vi "TcA03-003_MutualExclusionWhenModifyingClassAttributes.vi"(1 "Input buffer":T3="1", 3 "Invocation info":T2, 5 "error in (no error)":errorcluster, 6 "Add log to result?":bool) -> (16 "Test Data":T1 {"Numeric Measurement" format="%.2f"}, 19 "error out":errorcluster)   [LabVIEW 2020]
doc: "Test case template."
uses:
  Shared/Support_InputBuffer.ctl
  Shared/Support_InvocationInfo.ctl
  Shared/Support_TestData.ctl
  TestClasses/G#BaseClass1_class/G#BaseClass1.lvclass
  TestClasses/G#BaseClass2_class/G#BaseClass2.lvclass
  <vilib>/addons/_AddQ/G#Object/G#Object.lvclass
  TestClasses/G#SubClass2_class/G#SubClass2.lvclass
  TestClasses/G#SubClass1_class/G#SubClass1.lvclass
panel:
  in  "Test name":string="TcA03-003 Mutual Exclusion When Modifying Class Attributes"
  out "Test result":bool
  out "Result":string
  # "Verify that class attributes can be modified and\naccessed , one will be mutual excluded\nand forced to wait."
  # "Sub test case"
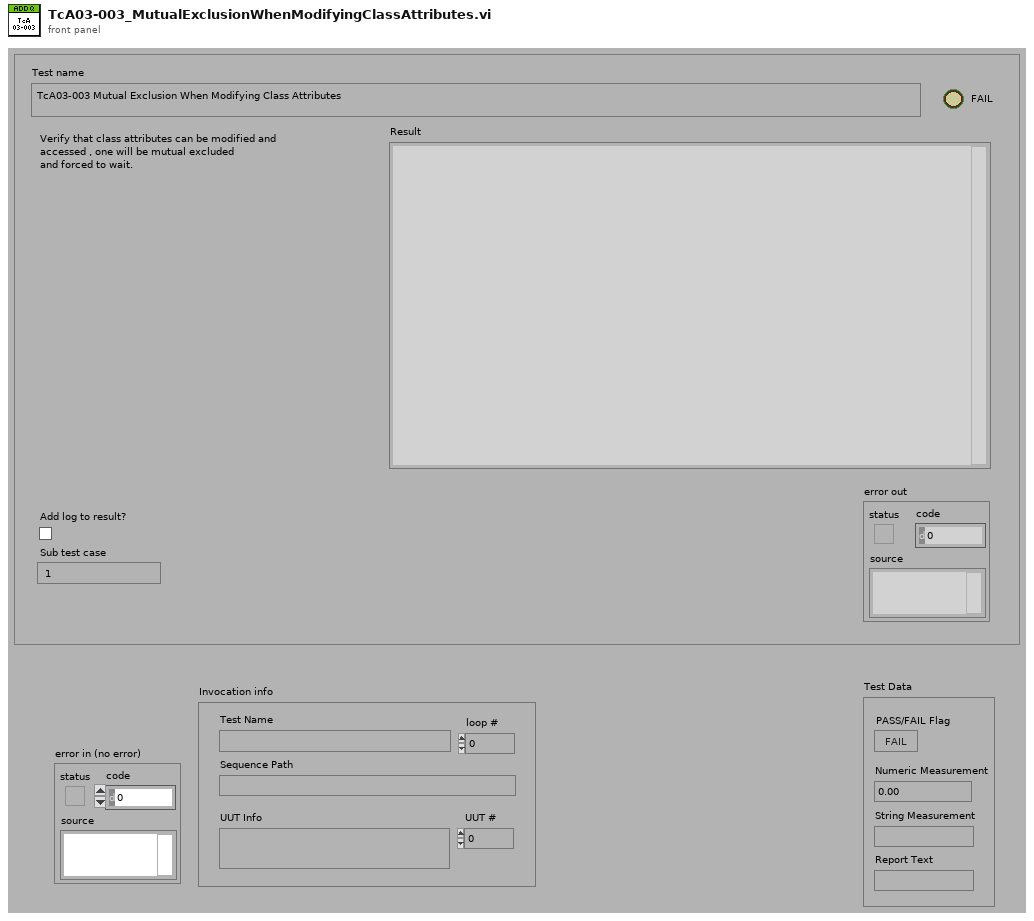
[diagram p1: front panel]
types:
  T1 = typedef "Support_TestData.ctl" = cluster{"PASS/FAIL Flag":bool, "Numeric Measurement":dbl, "String Measurement":string, "Report Text":string}
  T2 = typedef "Support_InvocationInfo.ctl" = cluster{"UUT #":i32, "loop #":i32, "UUT Info":string, "Test Name":string, "Sequence Path":path}
  T3 = typedef "Support_InputBuffer.ctl" = string
  T4 = typedef "Support_ResultType.ctl" = cluster{"Pass":bool, "Comment":string, "MeasurementValue":dbl}
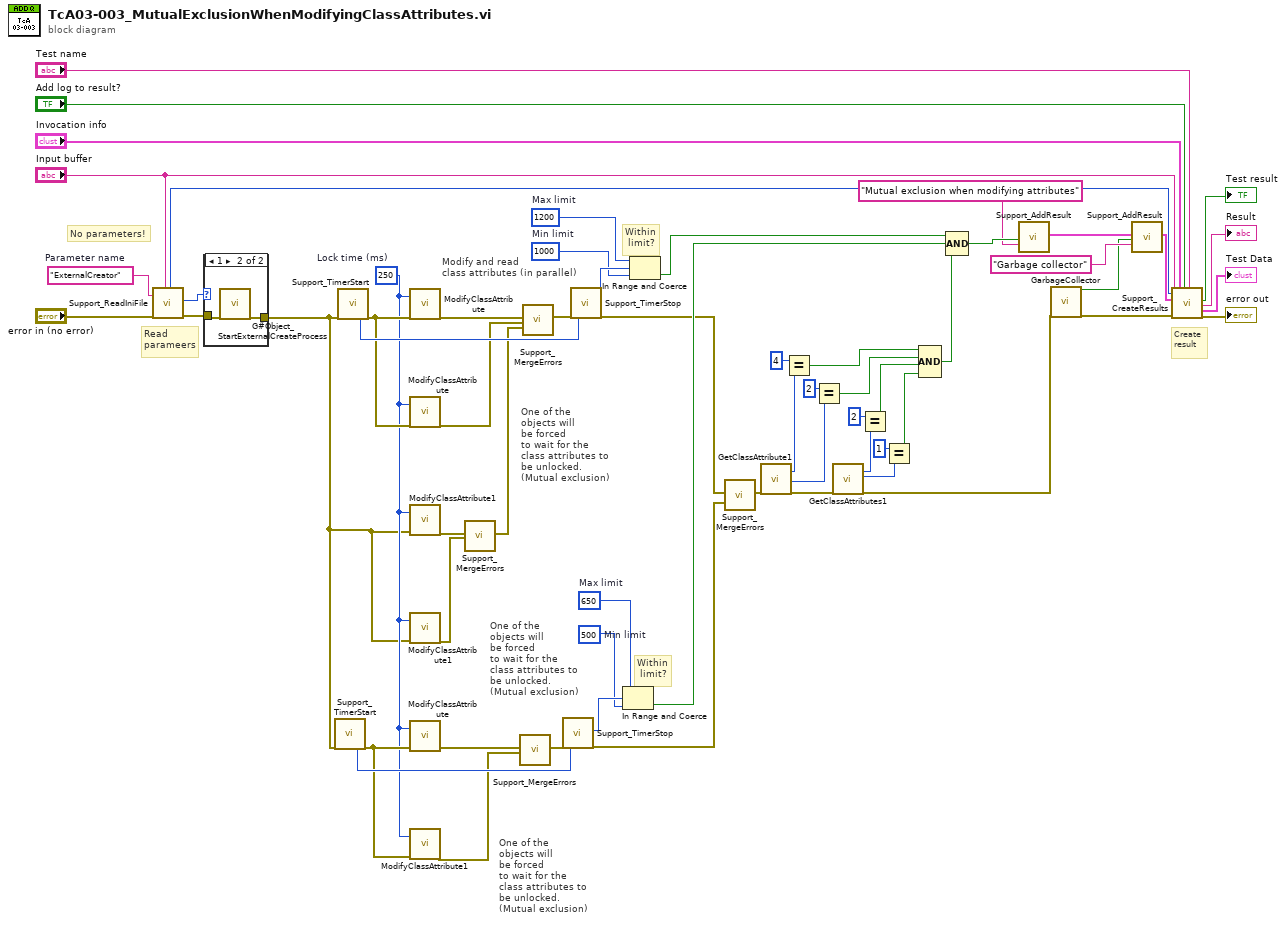
[diagram p0: block diagram]
diagram:
  w4 = "ExternalCreator"  # Parameter name
  w18 = u32 500  # Min limit
  w19 = u32 650  # Max limit
  w38 = u32 1000  # Min limit
  w39 = u32 1200  # Max limit
  w28 = u32 250  # Lock time (ms)
  # "Within\n limit?"
  # "One of the\nobjects will\nbe forced\nto wait for the\nclass attributes to\nbe unlocked.\n(Mutual exclusion)"
  # "One of the\nobjects will\nbe forced\nto wait for the\nclass attributes to\nbe unlocked.\n(Mutual exclusion)"
  # "One of the\nobjects will\nbe forced\nto wait for the\nclass attributes to\nbe unlocked.\n(Mutual exclusion)"
  # "Within\n limit?"
  # "Modify and read\nclass attributes (in parallel)"
  # "No parameters!"
  # "Create\nresult"
  # "Read\nparameers"
  n1 = call "Support_ReadIniFile.vi"("Parameter name"=w4, "error in (no error)"="error in (no error)", "Sub test case"="Input buffer") -> ("Timer start"=w52:u32, "Parameter1 as I32"=w1:i32, "error out"=w3:errorcluster)  [unwired: 9 in, 5 out]
  n2 = case shown="1" w1 {
    tunnel: w3 -> [w62 w64]
    tunnel: [w62 w63] -> w2
    frame 0, Default {
    }
    frame 1 {
      n3 = call <vilib>:"G#Object_StartExternalCreateProcess.vi"("error in (no error)"=w64) -> ("error out"=w63:errorcluster)  [unwired: 18 in]
    }
  }
  n4 = call "Support_TimerStart.vi"("error in (no error)"=w2) -> ("Start time"=w44:u32, "error out"=w41:errorcluster)  [unwired: 17 in]
  n5 = call "Support_TimerStart.vi"("error in (no error)"=w2) -> ("Start time"=w48:u32, "error out"=w42:errorcluster)  [unwired: 17 in]
  n6 = call "ModifyClassAttribute.vi"("Lock time (ms)"=w28, "error in (no error)"=w42) -> ("error out"=w50:errorcluster)  [unwired: 16 in, 1 out]
  n7 = call "ModifyClassAttribute.vi"("Lock time (ms)"=w28, "error in (no error)"=w42) -> ("error out"=w27:errorcluster)  [unwired: 16 in, 1 out]
  n8 = call "ModifyClassAttribute1.vi"("Lock time (ms)"=w28, "error in (no error)"=w2) -> ("error out"=w45:errorcluster)  [unwired: 17 in]
  n9 = call "ModifyClassAttribute1.vi"("Lock time (ms)"=w28, "error in (no error)"=w2) -> ("error out"=w26:errorcluster)  [unwired: 17 in]
  n10 = call "ModifyClassAttribute.vi"("Lock time (ms)"=w28, "error in (no error)"=w41) -> ("error out"=w47:errorcluster)  [unwired: 15 in, 2 out]
  n11 = call "ModifyClassAttribute1.vi"("Lock time (ms)"=w28, "error in (no error)"=w41) -> ("error out"=w25:errorcluster)  [unwired: 15 in, 2 out]
  n12 = call "Support_MergeErrors.vi"("error in 1"=w45, "error in 2"=w26) -> ("error out"=w20:errorcluster)  [unwired: 16 in, 1 out]
  n13 = call "Support_MergeErrors.vi"("error in 1"=w47, "error in 2"=w25) -> ("error out"=w46:errorcluster)  [unwired: 16 in, 1 out]
  n14 = call "Support_MergeErrors.vi"("error in 1"=w50, "error in 2"=w27, "error in 3"=w20) -> ("error out"=w49:errorcluster)  [unwired: 15 in, 1 out]
  n15 = call "Support_TimerStop.vi"("error in (no error)"=w46, "Start time"=w44) -> ("Time (ms)"=w37:u32, "error out"=w35:errorcluster)  [unwired: 16 in]
  n16 = call "Support_TimerStop.vi"("error in (no error)"=w49, "Start time"=w48) -> ("Time (ms)"=w40:u32, "error out"=w21:errorcluster)  [unwired: 16 in]
  n17 = In Range and Coerce(upper limit=w19, x=w37, lower limit=w18) -> (In Range?=w34:bool)  [unwired: 1 out]
  n18 = In Range and Coerce(upper limit=w39, x=w40, lower limit=w38) -> (In Range?=w36:bool)  [unwired: 1 out]
  n19 = call "Support_MergeErrors.vi"("error in 1"=w21, "error in 3"=w35) -> ("error out"=w24:errorcluster)  [unwired: 16 in, 1 out]
  n20 = call "GetClassAttribute1.vi"("error in (no error)"=w24) -> ("Int"=w17:i32, "SubClassIntAttribute"=w15:i32, "error out"=w23:errorcluster)  [unwired: 15 in, 1 out]
  n21 = Equal?(x=4, y=w17) -> (x = y?=w9:bool)
  n22 = Equal?(x=2, y=w15) -> (x = y?=w8:bool)
  n23 = call "GetClassAttributes1.vi"("error in (no error)"=w23) -> ("Base class.ClassAttr"=w13:i32, "SubClassAttr"=w11:i32, "error out"=w22:errorcluster)  [unwired: 15 in, 1 out]
  n24 = Equal?(x=2, y=w13) -> (x = y?=w7:bool)
  n25 = Equal?(x=1, y=w11) -> (x = y?=w6:bool)
  n26 = Compound Arithmetic op=AND(w9, w8, w7, w6) -> (w5:bool)
  n27 = Compound Arithmetic op=AND(w36, w34, w5) -> (w43:bool)
  n28 = call "Support_AddResult.vi"("Pass"=w43, "Comment"="Mutual exclusion when modifying attributes") -> ("Results out"=w32:T4[])  [unwired: 17 in]
  n29 = call <vilib>:"GarbageCollector.vi"("error in (no error)"=w22) -> ("OK"=w29:bool, "error out"=w51:errorcluster)  [unwired: 16 in, 1 out]
  n30 = call "Support_AddResult.vi"("Results in"=w32, "Pass"=w29, "Comment"="Garbage collector") -> ("Results out"=w31:T4[])  [unwired: 16 in]
  n31 = call "Support_CreateResults.vi"("Sub test case"="Input buffer", "Timer start"=w52, "Results"=w31, "error in (no error)"=w51, "Invocation info"="Invocation info", "Add log to result?"="Add log to result?", "Test name"="Test name") -> ("Pass/fail flag"=→"Test result":bool, "Result"=→"Result":string, "Test Data"=→"Test Data":T1, "error out"=→"error out":errorcluster)  [unwired: 9 in]
